vi "2_2_Temperatura.vi"() -> ()   [LabVIEW 2020]
uses:
  <vilib>/numeric/Random Number (Range) U64.vi
  <vilib>/numeric/sub_Random U32.vi
panel:
  in  "Alpha":dbl=0.1
  out "Grados °C":cluster{dbl[], u64[]}(graph)
  out "Tabla de Grados":dbl[][](array[numeric])
  in  "Cantidad de \ngrados a crear":i32
  # "centigrados"
  # "Farenheit"
  # "Filto EMA"
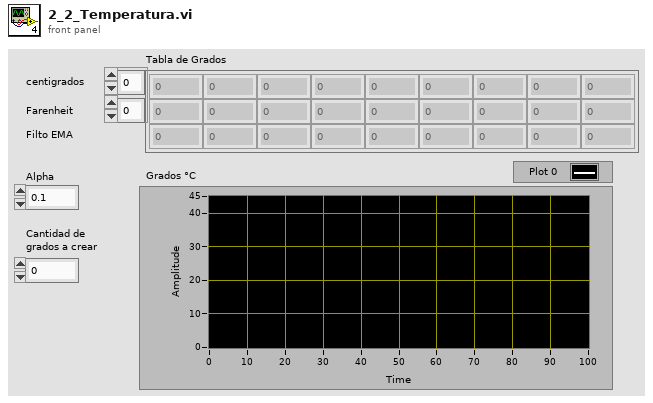
[diagram p1: front panel]
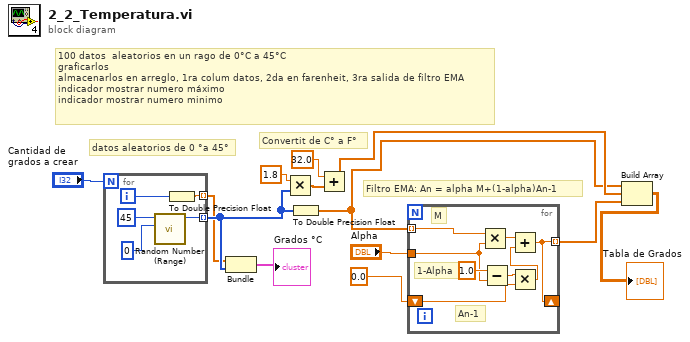
[diagram p0: block diagram]
diagram:
  # "Filtro EMA: An = alpha M+(1-alpha)An-1"
  # "Convertit de C° a F°"
  # "datos aleatorios de 0 °a 45°"
  # "100 datos  aleatorios en un rago de 0°C a 45°C\ngraficarlos\nalmacenarlos en arreglo, 1ra colum datos, 2da en farenheit, 3ra salida de filtro EMA\nindicador mostrar numero máximo\nindicador mostrar numero minimo"
  n1 = for {
    N: "Cantidad de \ngrados a crear" -> [_]
    tunnel: [w16] -> w9 mode=indexing
    tunnel: [w14] -> w8 mode=indexing
    i -> [w15]
    n2 = call-poly <vilib>:"Random Number (Range).vi"("lower bound (0)"=u64 0, "upper bound (100)"=u64 45) -> ("number"=w16:u64)  [unwired: 9 in]
    n3 = To Double Precision Float(number=w15) -> (double precision float=w14:dbl)
  }
  n4 = Bundle "Bundle"(w8, w9) -> (→"Grados °C":cluster{dbl[], u64[]})  [unwired: 1 in]
  n5 = Multiply(x=1.8, y=w9) -> (x*y=w1:dbl[])
  n6 = To Double Precision Float(number=w9) -> (double precision float=w5:dbl[])
  n7 = Add(x=32.0, y=w1) -> (x+y=w11:dbl[])
  n8 = for {
    tunnel: w5 -> [w25] mode=indexing
    shift-right: [w19] -> _
    shift-left: 0.0 -> [w23]
    tunnel: "Alpha" -> [w24]
    tunnel: [w19] -> w2 mode=indexing
    # "An-1"
    # "1-Alpha"
    # "M"
    n9 = Multiply(x=w25, y=w24) -> (x*y=w21:dbl)
    n10 = Subtract(x=1.0, y=w24) -> (x-y=w22:dbl)
    n11 = Multiply(x=w22, y=w23) -> (x*y=w20:dbl)
    n12 = Add(x=w21, y=w20) -> (x+y=w19:dbl)
  }
  n13 = Build Array "Build Array"(w5, w11, w2) -> (→"Tabla de Grados":dbl[][])
